vi "Get Sensor Data.vi"(8 "error in (no error)":errorcluster, 9 "Intercept":dbl, 10 "Slope":dbl, 11 "Sensor Parameter in":refnum<class "Sensor Parameter.lvclass">) -> (0 "error out":errorcluster, 3 "Sensor Parameter out":refnum<class "Sensor Parameter.lvclass">)   [LabVIEW 2013, in "Parameter.lvlib" / "Sensor Parameter.lvclass"]
uses:
  Sensor Parameter.lvclass
  Abstract Sensor Parameter/Abstract Sensor Parameter.lvclass/Abstract Sensor Parameter.ctl
  Abstract Sensor Parameter/Data Accessors/Set Value.vi
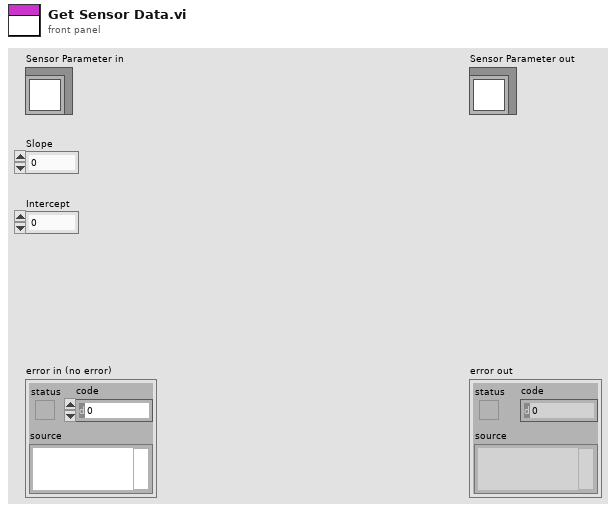
[diagram p1: front panel]
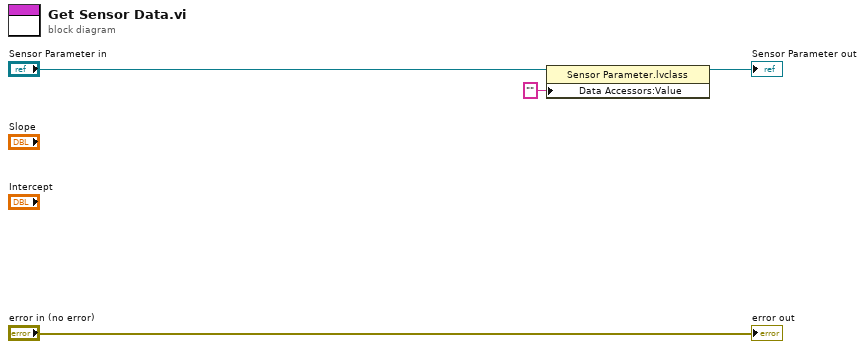
[diagram p0: block diagram]
diagram:
  n1 = property class="Sensor Parameter.lvclass"(reference="Sensor Parameter in", "Data Accessors:Value"="" ("Value")) -> (reference out=→"Sensor Parameter out":refnum<class "Sensor Parameter.lvclass">)  [unwired: 1 in, 1 out]
  "error out" <- "error in (no error)"
